vi "RxTestExample.vi"() -> ()   [LabVIEW 2015, in "QCA_DUT_Func.lvlib"]
uses:
  QCA_DUT_Func.lvlib
panel:
  out "return type 2":u8
  in  "Cluster":T1={"channel"=5180, "channel2"=5290, "rxMode"=0, "rxChain"=1, "wlanMode"=8, "rateMask"=60, "antenna"=0, "bandwidth"=0}
  out "return type":u8=1
  out "goodPackets":i32
  in  "Bin_file":string="D:\\4-Up-WLAN-Test-System\\board_data\\boardData_QCA9984_CUS239_5G_v1_001.bin"
  in  "chip_select":i32=3
  in  "DUT_IP":string="192.168.1.2"
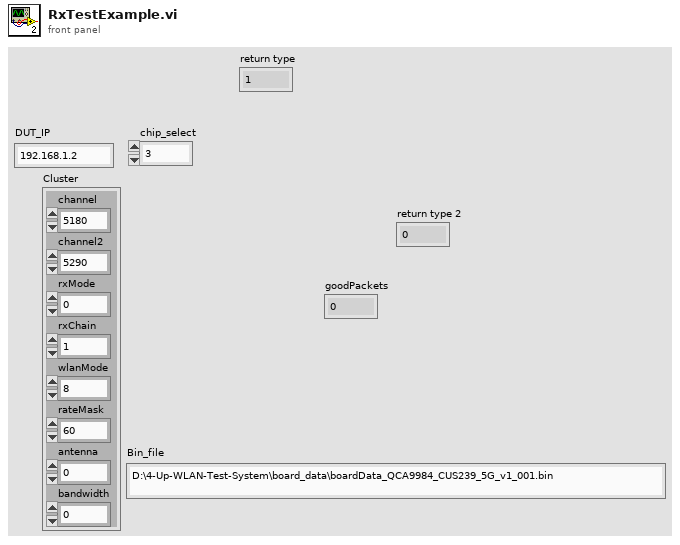
[diagram p1: front panel]
types:
  T1 = cluster{"channel":u32, "channel2":u32, "rxMode":u32, "rxChain":u32, "wlanMode":u32, "rateMask":u32, "antenna":u32, "bandwidth":u32}
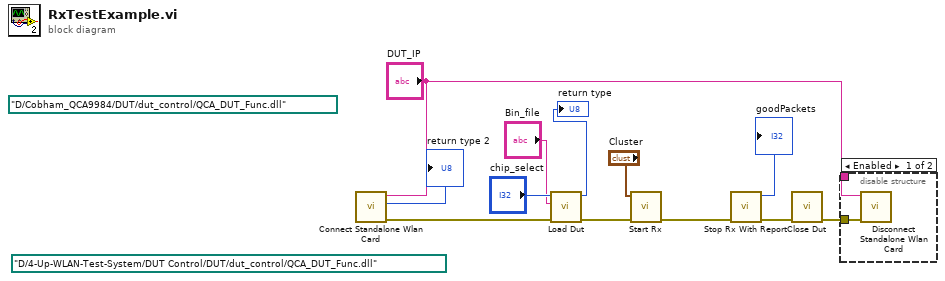
[diagram p0: block diagram]
diagram:
  (unwired) path "D:/4-Up-WLAN-Test-System/DUT Control/DUT/dut_control/QCA_DUT_Func.dll" ("path in")
  (unwired) path "D:/Cobham_QCA9984/DUT/dut_control/QCA_DUT_Func.dll" ("path in")
  n1 = call "Connect Standalone Wlan Card.vi"("DUT_IP"="DUT_IP") -> ("error out"=w12:errorcluster, "return type"=→"return type 2":u8)  [unwired: 8 in, 1 out]
  n2 = call "Load Dut.vi"("error in (no error)"=w12, "Bin_file"="Bin_file", "chip_select"="chip_select") -> ("error out"=w7:errorcluster, "return type"=→"return type":u8)  [unwired: 6 in, 1 out]
  n3 = call "Start Rx.vi"("error in (no error)"=w7, "Cluster"="Cluster") -> ("error out"=w3:errorcluster)  [unwired: 9 in]
  n4 = call "Stop Rx With Report.vi"("error in (no error)"=w3) -> ("error out"=w2:errorcluster, "return type"=→"goodPackets":i32)  [unwired: 9 in]
  n5 = call "Close Dut.vi"("error in (no error)"=w2) -> ("error out"=w9:errorcluster)  [unwired: 10 in]
  n6 = disable-structure shown="Enabled" {
    disable-tunnel: w9 -> [w14 _]
    disable-tunnel: "DUT_IP" -> [w13 _]
    frame Enabled {
      n7 = call "Disconnect Standalone Wlan Card.vi"("error in (no error)"=w14, "DUT_IP"=w13) -> ()  [unwired: 8 in, 2 out]
    }
    frame Disabled {
    }
  }
